vi "Variant to Syringe Event.vi"(8 "error in (no error)":errorcluster, 10 "variant":variant, 11 "Syringe in":refnum<class "Syringe.lvclass">) -> (0 "error out":errorcluster, 2 "Event Registration Refnum":refnum<event-registration>, 3 "Syringe out":refnum<class "Syringe.lvclass">)   [LabVIEW 2015, in "AMS UI.lvlib" / "Syringe.lvclass"]
uses:
  Syringe.lvclass
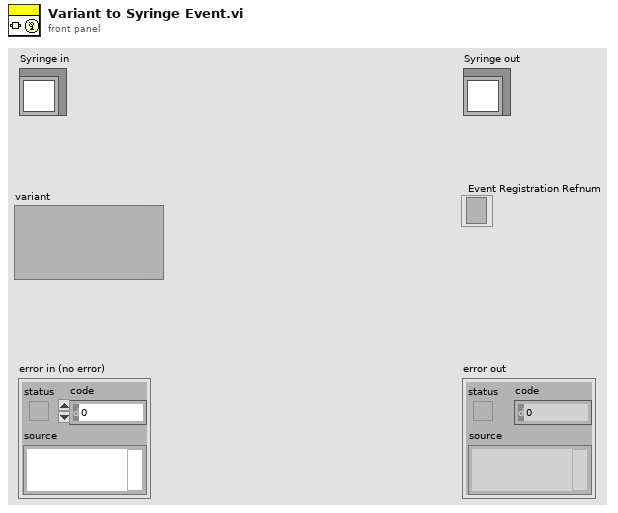
[diagram p1: front panel]
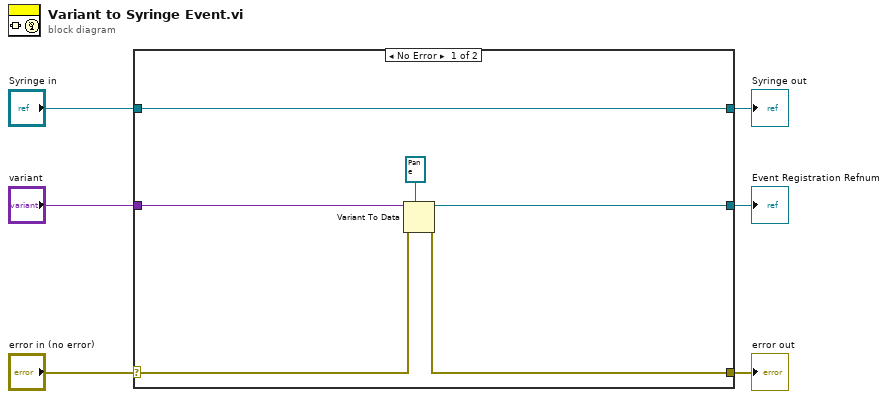
[diagram p0: block diagram]
diagram:
  n1 = case shown="No Error" "error in (no error)" {
    selector: "error in (no error)" -> [w10 w14]
    tunnel: [w9 w14] -> w5
    tunnel: [w12 w13] -> w3
    tunnel: "Syringe in" -> [w12 w13]
    tunnel: "variant" -> [w11 _]
    tunnel: [w7 _] -> w1
    frame No Error {
      n2 = Variant To Data(error in=w10, type=refnum<event-registration> refnum ("event registration refnum"), Variant=w11) -> (data=w7:refnum<event-registration>, error out=w9:errorcluster)
    }
    frame Error {
    }
  }
  "error out" <- w5
  "Syringe out" <- w3
  "Event Registration Refnum" <- w1
